vi "Util_TrajState_to_DiffDrive_WheelPos.vi"(9 "Wheelbase":dbl, 11 "TRAJ_STATE":T1={"TimeSeconds"=0.0, "Velocity"=0.0, "Acceleration"=0.0, "POSE"={"TRANSLATION"={"X"=0.0, "Y"=0.0}, "ROTATION"={"VALUE"=0.0, "COS"=1.0, "SIN"=0.0}}, "Curvature"=0.0} {"POSE"."ROTATION"."SIN" format="%13.4f"; "POSE"."ROTATION"."COS" format="%13.4f"; "POSE"."ROTATION"."VALUE" format="%13.4f"; "POSE"."TRANSLATION"."Y" format="%14.3f"; "POSE"."TRANSLATION"."X" format="%14.3f"}) -> (0 "Right Y":dbl, 1 "Right X":dbl, 2 "Left Y":dbl, 3 "Left X":dbl)   [LabVIEW 2019, in "Trajectory_Library.lvlib"]
doc: "Utility function to create the position of individual differential drive wheels from a trajectory state. This is used to plot the wheel positions. Inputs are Meters and Radians"
uses:
  Trajectory_Library.lvlib
  TypeDef/TRANSLATION2D.ctl
  TypeDef/ROTATION2D.ctl
  TypeDef/POSE2D.ctl
  TypeDef/TRAJ_STATE.ctl
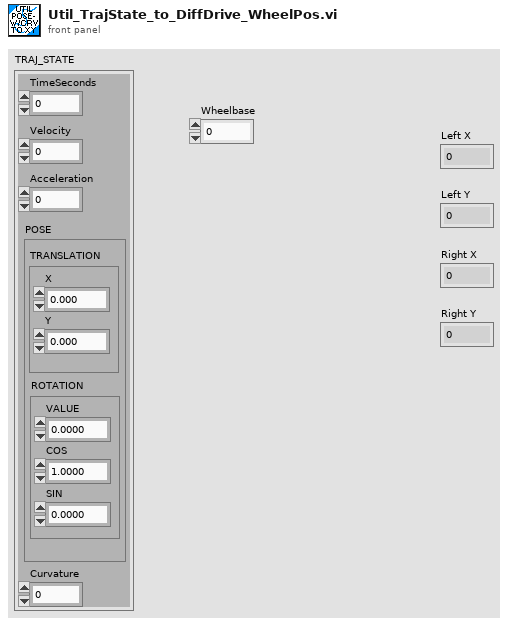
[diagram p1: front panel]
types:
  T1 = typedef "Trajectory_Library.lvlib/TRAJ_STATE.ctl" = cluster{"TimeSeconds":dbl, "Velocity":dbl, "Acceleration":dbl, "POSE":T2, "Curvature":dbl}
  T2 = typedef "Trajectory_Library.lvlib/POSE2D.ctl" = cluster{"TRANSLATION":T3, "ROTATION":T4}
  T3 = typedef "Trajectory_Library.lvlib/TRANSLATION2D.ctl" = cluster{"X":dbl, "Y":dbl}
  T4 = typedef "Trajectory_Library.lvlib/ROTATION2D.ctl" = cluster{"VALUE":dbl, "COS":dbl, "SIN":dbl}
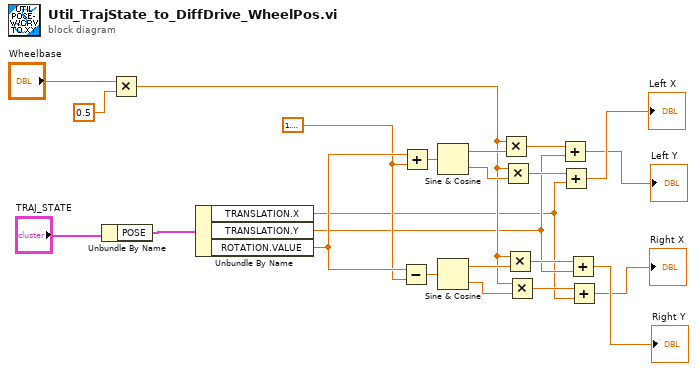
[diagram p0: block diagram]
diagram:
  w9 = 1.5707963267948966
  n1 = Unbundle By Name("TRAJ_STATE") -> ("POSE"=w23:T2)
  n2 = Multiply(x="Wheelbase", y=0.5) -> (x*y=w8:dbl)
  n3 = Unbundle By Name(w23) -> ("TRANSLATION.X"=w6:dbl, "TRANSLATION.Y"=w7:dbl, "ROTATION.VALUE"=w10:dbl)
  n4 = Subtract(x=w10, y=w9) -> (x-y=w15:dbl)
  n5 = Add(x=w10, y=w9) -> (x+y=w20:dbl)
  n6 = Sine & Cosine(0:w20) -> (1:w18:dbl, 2:w19:dbl)
  n7 = Sine & Cosine(0:w15) -> (1:w13:dbl, 2:w14:dbl)
  n8 = Multiply(x=w8, y=w18) -> (x*y=w16:dbl)
  n9 = Multiply(x=w8, y=w19) -> (x*y=w17:dbl)
  n10 = Multiply(x=w8, y=w13) -> (x*y=w11:dbl)
  n11 = Multiply(x=w8, y=w14) -> (x*y=w12:dbl)
  n12 = Add(x=w16, y=w7) -> (x+y=→"Left Y":dbl)
  n13 = Add(x=w17, y=w6) -> (x+y=→"Left X":dbl)
  n14 = Add(x=w11, y=w7) -> (x+y=→"Right Y":dbl)
  n15 = Add(x=w12, y=w6) -> (x+y=→"Right X":dbl)
